vi "byteToHex.vi"(1 "Byte string":string) -> (0 "hex integer string":string)   [LabVIEW 2015]
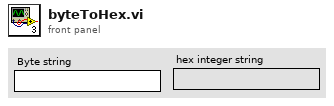
[diagram p1: front panel]
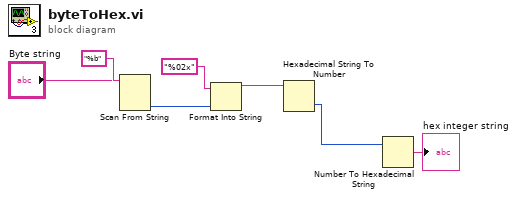
[diagram p0: block diagram]
diagram:
  n1 = Scan From String(format string="%b", input string="Byte string") -> (output 1=w6:i32)  [unwired: 3 in, 3 out]
  n2 = Format Into String(format string="%02x", w6) -> (resulting string=w3:string)  [unwired: 2 in, 1 out]
  n3 = Hexadecimal String To Number(string=w3) -> (number=w2:u32)  [unwired: 2 in, 1 out]
  n4 = Number To Hexadecimal String(2:w2) -> (0:→"hex integer string":string)  [unwired: 1 in]
